vi "Data Display Loop.vi"(10 "Message Queues in":T1, 11 "WaveformChart in":refnum<vi>) -> ()   [LabVIEW 2018]
uses:
  Message Queue/All Message Queues.ctl
  Message Queue/Message Cluster.ctl
  Controls/Data Queue.ctl
  Controls/Acquired Data.ctl
  Controls/Data Notifier.ctl
  Message Queue/Message Queue.lvlib
panel:
  out "error out":errorcluster
  in  "error in (no error)":errorcluster
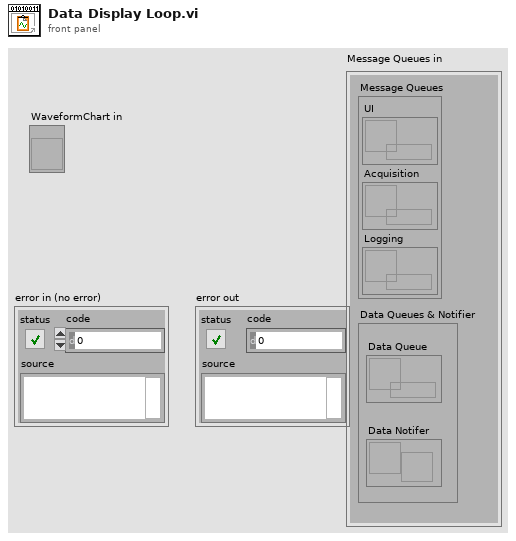
[diagram p1: front panel]
types:
  T1 = typedef "Message Queue.lvlib/All Message Queues.ctl" = cluster{"Message Queues":cluster{"UI":refnum<queue>, "Acquisition":refnum<queue>, "Logging":refnum<queue>}, "Data Queues & Notifier":cluster{"Data Queue":T2, "Data Notifer":T3}}
  T2 = typedef "Data Queue.ctl" = refnum<queue>
  T3 = typedef "Data Notifier.ctl" = refnum<notifier>
  T4 = typedef "Acquired Data.ctl" = cluster{"offset":dbl, "time":string}
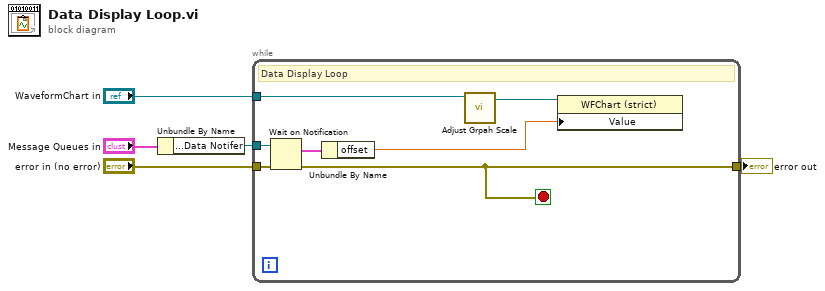
[diagram p0: block diagram]
diagram:
  n1 = Unbundle By Name("Message Queues in") -> ("Data Queues & Notifier.Data Notifer"=w1:T3)
  n2 = while "Data Display Loop" {
    tunnel: "WaveformChart in" -> [w11]
    tunnel: w1 -> [w10]
    tunnel: "error in (no error)" -> [w9]
    tunnel: [w8] -> w3
    stop <- w8 stop-if-true
    # "Data Display Loop"
    n3 = Wait on Notification(notifier=w10, error in (no error)=w9) -> (notification=w12:T4, error out=w8:errorcluster)  [unwired: 2 in, 2 out]
    n4 = Unbundle By Name(w12) -> ("offset"=w6:dbl)
    n5 = call "Adjust Grpah Scale.vi"("WaveformChart in"=w11) -> ("WaveformChart out"=w7:refnum<vi>)  [unwired: 10 in]
    n6 = property class="WFChart (strict)"(reference=w7, "Value"=w6) -> ()  [unwired: 1 in, 2 out]
  }
  "error out" <- w3
